vi "Write ShortTestReport.vi"(8 "error in (no error)":errorcluster, 10 "ShortTestReport":string[](array[string]), 11 "TestBench in":refnum<class "TestBench.lvclass">) -> (0 "error out":errorcluster, 3 "TestBench out":refnum<class "TestBench.lvclass">)   [LabVIEW 2019, in "TestBench.lvlib" / "TestBench.lvclass"]
uses:
  TestBench.lvclass
  <vilib>/addons/database/Auxilliary.llb/DB Tools Column Info.ctl
  <vilib>/addons/database/Auxilliary.llb/DB Tools DataTypes.ctl
  TestBench.lvclass/TestBench.ctl
  DataBase/DataBase Messages/WriteData Msg/WriteData Msg.lvclass/WriteData Msg.ctl
  <vilib>/ActorFramework/Message Enqueuer/Message Enqueuer.lvclass/Message Enqueuer.ctl
  <vilib>/ActorFramework/Message Enqueuer/Enqueue.vi
  DataBase/DataBase Messages/WriteData Msg/WriteData Msg.lvclass
  C:/Program Files (x86)/National Instruments/LabVIEW 2019/vi.lib/ActorFramework/Message/Message.lvclass
  <vilib>/ActorFramework/Message Priority Queue/Priority Enqueue.vi
  <vilib>/addons/database/NI_Database_API.lvlib
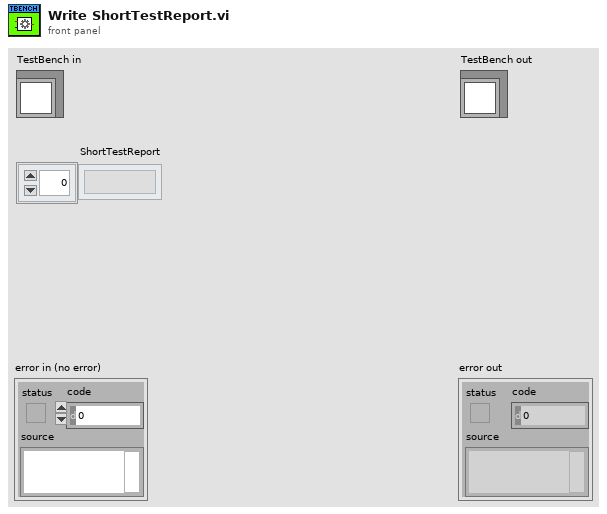
[diagram p1: front panel]
types:
  T1 = typedef "NI_Database_API.lvlib/DB Tools Column Info.ctl" = cluster{"column name":string, "data type":T2, "size":i32, "allow null?":bool}
  T2 = typedef "NI_Database_API.lvlib/DB Tools DataTypes.ctl" = enum16{"String", "Long (I32)", "Single (SGL)", "Double (DBL)", "Date/Time", "Binary"}
  T3 = enum16{"Station 1", "Station 2", "Station 3", "Station 4"}
  T4 = cluster{"ShortTestReport[0]":string, "ShortTestReport[1]":string, "ShortTestReport[2]":string, "ShortTestReport[3]":string}
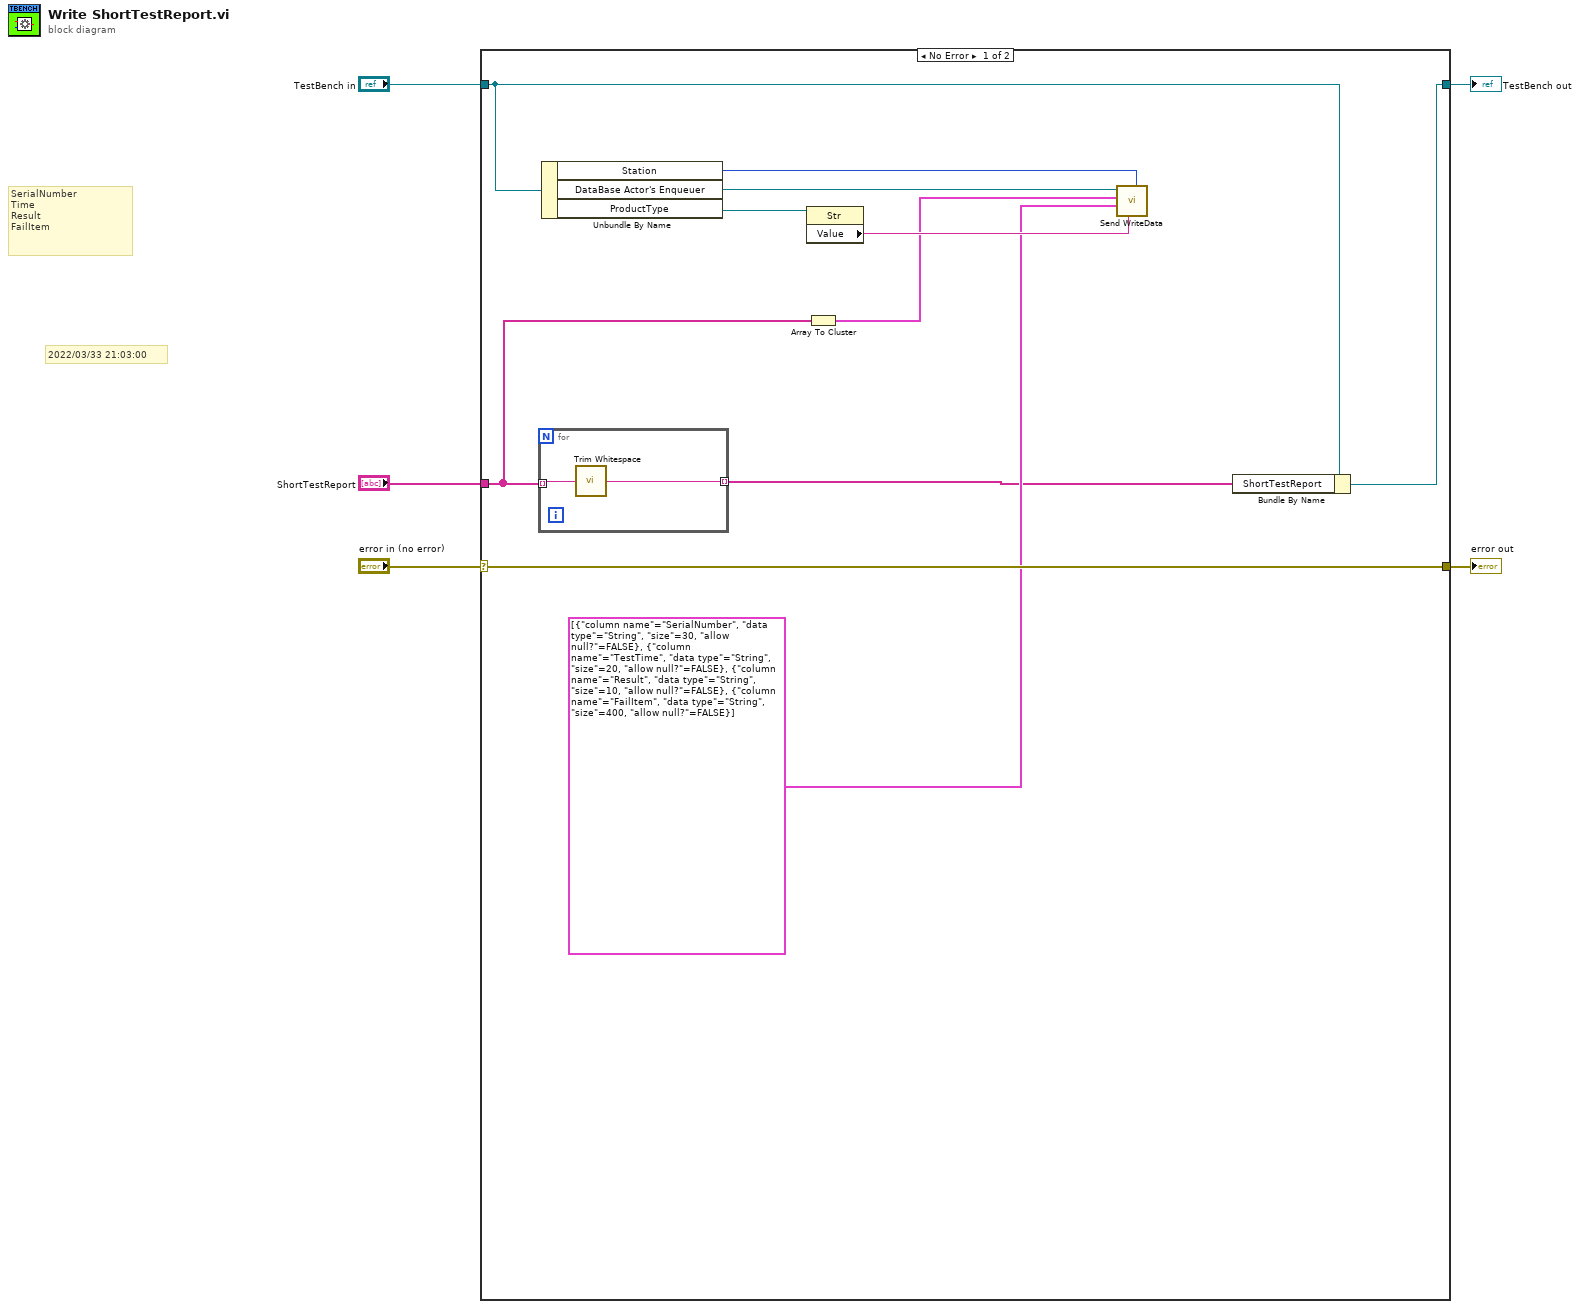
[diagram p0: block diagram]
diagram:
  # "2022/03/33 21:03:00"
  # "SerialNumber\nTime\nResult\nFailItem"
  n1 = case shown="No Error" "error in (no error)" {
    selector: "error in (no error)" -> [w16 w19]
    tunnel: [w16 w19] -> w4
    tunnel: [w15 w20] -> w2
    tunnel: "TestBench in" -> [w14 w20]
    tunnel: "ShortTestReport" -> [w7 _]
    frame No Error {
      n2 = for {
        tunnel: w7 -> [w18] mode=indexing
        tunnel: [w17] -> w9 mode=indexing
        n3 = call <vilib>:"Trim Whitespace.vi"("string"=w18) -> ("trimmed string"=w17:string)  [unwired: 1 in]
      }
      n4 = Unbundle By Name(w14) -> ("Station"=w6:T3, "DataBase Actor's Enqueuer"=w12:refnum<class "Message Enqueuer.lvclass">, "ProductType"=w13:refnum<vi>)
      n5 = property class="Str"(reference=w13) -> ("Value"=w11:string)  [unwired: 1 in, 2 out]
      n6 = Array To Cluster(array=w7) -> (cluster=w8:T4)
      n7 = call "Send WriteData.vi"("Station"=w6, "TableName"=w11, "column information"=T1[] [{"column name"="SerialNumber", "data type"=enum."String", "size"=30, "allow null?"=FALSE}, {"column name"="TestTime", "data type"=enum."String", "size"=20, "allow null?"=FALSE}, {"column name"="Result", "data type"=enum."String", "size"=10, "allow null?"=FALSE}, {"column name"="FailItem", "data type"=enum."String", "size"=400, "allow null?"=FALSE}], "data"=w8, "Message Enqueuer"=w12) -> ()  [unwired: 5 in, 2 out]
      n8 = Bundle By Name(cluster=w14, "ShortTestReport"=w9) -> (w15:refnum<class "TestBench.lvclass">)
    }
    frame Error {
    }
  }
  "error out" <- w4
  "TestBench out" <- w2
